vi "LINC Read Packet Configuration.vi"(8 "error in (no error)":errorcluster, 9 "packet name":string, 10 "type":enum16{"CMD", "TLM"}(ring), 11 "LINC session":refnum<class "LINC.lvclass">) -> (0 "error out":errorcluster, 1 "item formats":T1[](array[typedef]), 2 "item names":string[](array[string]), 3 "dup LINC session":refnum<class "LINC.lvclass">)   [LabVIEW 2018, in "STEPkgDriver_LINC.lvlib" / "LINC.lvclass"]
uses:
  LINC.lvclass
  LINC Global Mode.ctl
  STEPkgDriver_LINC.lvlib
  LINC Format Prototype.ctl
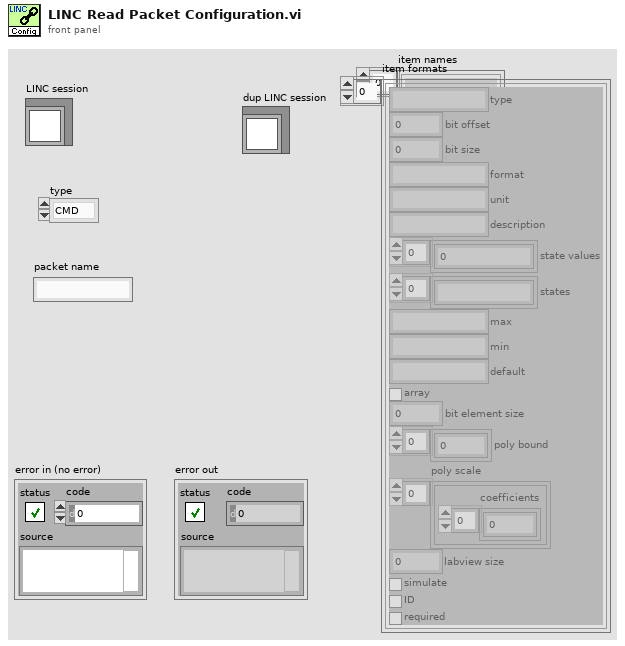
[diagram p1: front panel]
types:
  T1 = typedef "STEPkgDriver_LINC.lvlib/LINC Format Prototype.ctl" = cluster{"type":string, "bit offset":i32, "bit size":i32, "format":string, "unit":string, "description":string, "state values":i64[], "states":string[], "max":string, "min":string, "default":string, "array":bool, "bit element size":i32, "poly bound":dbl[], "poly scale":cluster{"coefficients":dbl[]}[], "labview size":i32, "simulate":bool, "ID":bool, "required":bool}
  T2 = typedef "STEPkgDriver_LINC.lvlib/LINC Global Mode.ctl" = enum16{"INIT", "CLEAR", "ADD_PKT_HDR", "ADD_PKT", "GET_PKT_NAMES", "GET_PKT_DESC", "GET_PKT_HDR", "GET_PKT", "SET_PKT", "SET_DATA", "SIM_EN", "SIM_DS"}
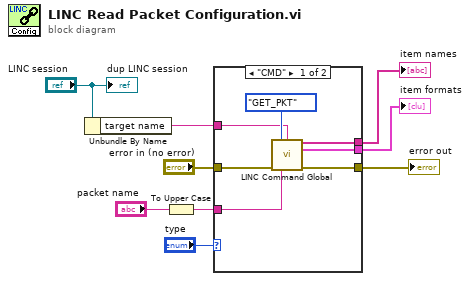
[diagram p0: block diagram]
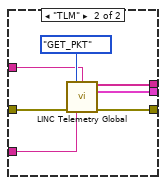
[diagram p2: hidden frame]
diagram:
  n1 = Unbundle By Name("LINC session") -> ("target name"=w7:string)
  n2 = To Upper Case(1:"packet name") -> (0:w1:string)
  n3 = case shown="\"CMD\"" "type" {
    tunnel: "error in (no error)" -> [w15 w22]
    tunnel: [w14 w21] -> w8
    tunnel: w7 -> [w13 w20]
    tunnel: w1 -> [w12 w19]
    tunnel: [w11 w18] -> w4
    tunnel: [w10 w17] -> w3
    frame "CMD" {
      n4 = call "LINC Command Global.vi"("mode"=LINC_Global_Mode."GET_PKT", "target name"=w13, "error in (no error)"=w15, "packet name"=w12) -> ("values out"=w11:string[], "item formats out"=w10:T1[], "error out"=w14:errorcluster)  [unwired: 7 in, 2 out]
    }
    frame "TLM" {
      n5 = call "LINC Telemetry Global.vi"("mode"=LINC_Global_Mode."GET_PKT", "target name"=w20, "error in (no error)"=w22, "packet name"=w19) -> ("values out"=w18:string[], "item formats out"=w17:T1[], "error out"=w21:errorcluster)  [unwired: 7 in, 2 out]
    }
  }
  "error out" <- w8
  "item names" <- w4
  "item formats" <- w3
  "dup LINC session" <- "LINC session"
